vi "Read Measurement (Switching Loss Power Analysis).vi"(0 "VISA resource name":refnum<visa-resource-name>, 5 "Switching Loss Measurement Type (0: Energy Loss)":i32(ring) items=["Energy Loss", "Power Loss", "Power Loss Per Cycle"], 11 "error in (no error)":errorcluster) -> (4 "VISA resource name out":refnum<visa-resource-name>, 6 "Switching Loss Measurement":dbl, 15 "error out":errorcluster)   [LabVIEW 2017, in "Agilent 2000 3000 X-Series.lvlib"]
doc: "Returns the measurement of a switching loss power analysis.\n\n<B>Note(s):</B>\nUse <B>Configure Power Analysis (Switching Loss).vi</B> to apply a power analysis.\nThis VI is not supported by EDUX1052A/G, DSOX1202A/G, DSOX1204A/G models"
uses:
  Agilent 2000 3000 X-Series.lvlib
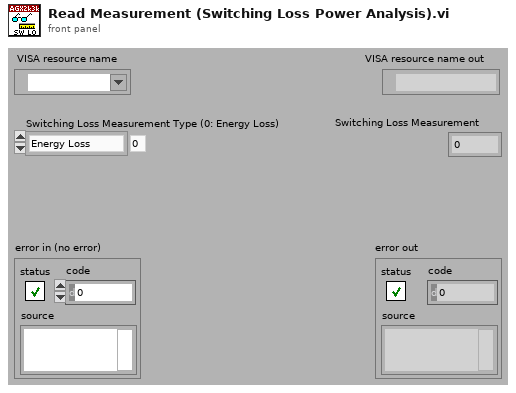
[diagram p1: front panel]
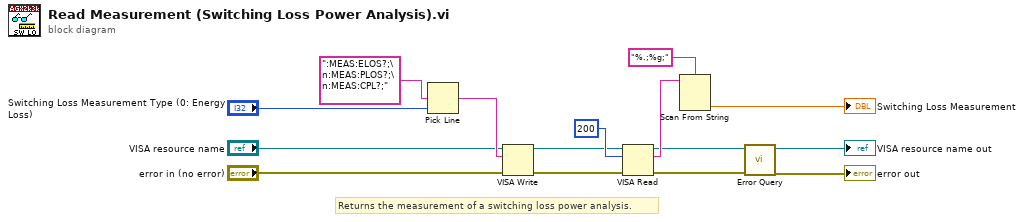
[diagram p0: block diagram]
diagram:
  # "Returns the measurement of a switching loss power analysis."
  n1 = Pick Line(multi-line string=":MEAS:ELOS?;\n:MEAS:PLOS?;\n:MEAS:CPL?;", line index="Switching Loss Measurement Type (0: Energy Loss)") -> (output string=w13:string)  [unwired: 1 out]
  n2 = VISA Write(VISA resource name="VISA resource name", write buffer=w13, error in (no error)="error in (no error)") -> (VISA resource name out=w6:refnum<visa-resource-name>, error out=w5:errorcluster)  [unwired: 1 out]
  n3 = VISA Read(VISA resource name=w6, byte count=u32 200, error in (no error)=w5) -> (VISA resource name out=w3:refnum<visa-resource-name>, read buffer=w7:string, error out=w4:errorcluster)  [unwired: 1 out]
  n4 = Scan From String(format string="%.;%g;", input string=w7) -> (output 1=→"Switching Loss Measurement":dbl)  [unwired: 2 in, 4 out]
  n5 = call "Error Query.vi"("error in (no error)"=w4, "VISA resource name"=w3) -> ("error out"=→"error out":errorcluster, "VISA resource name out"=→"VISA resource name out":refnum<visa-resource-name>)  [unwired: 8 out]
